vi "Solve Band Linear Equations (multiple right hand).vi"(8 "Known Vectors":T1, 9 "# of super-diagonal":i32, 10 "# of sub-diagonal":i32, 11 "Banded Matrix":dbl[][](array[numeric]) format="%.2f") -> (0 "error":i32, 3 "Solution Vectors":T1)   [LabVIEW 2017, in "NI_AALPro.lvlib"]
doc: "Computes the solution to the system of linear equations AX=Y with a band coefficient matrix A and single or multiple right-hand sides Y."
uses:
  NI_AALPro.lvlib
  RealMatrix.ctl
  lvanlys.dll
  NI_Matrix.lvlib
panel:
  # "Solve Band Linear Equations"
  # "Must be in band storage"
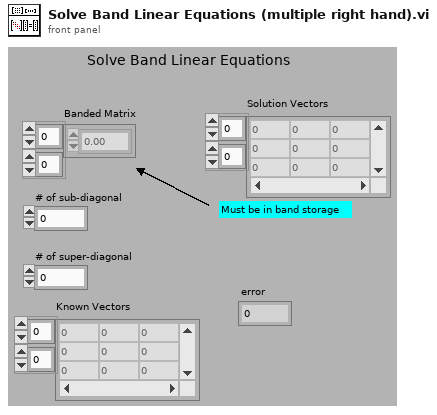
[diagram p1: front panel]
types:
  T1 = typedef "NI_Matrix.lvlib/RealMatrix.ctl" = dbl[][]
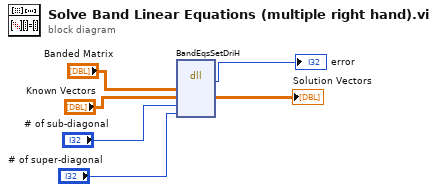
[diagram p0: block diagram]
diagram:
  n1 = dll-call lib="C:/Program Files/National Instruments/LabVIEW 2017/resource/lvanlys.*" fn="BandEqsSetDriH"("Banded Matrix"="Banded Matrix", "Known Vectors"="Known Vectors", "kl"="# of sub-diagonal", "ku"="# of super-diagonal") -> (→"error":i32, "Known Vectors"=→"Solution Vectors":T1)  [unwired: 6 in, 2 out]
